vi "PmSetReadoutMode.vi"(8 "error in (no error)":errorcluster, 10 "Readout Mode":T1(ring)=enum."Speed (8-bit)", 11 "Camera in":refnum<class "Camera.lvclass">) -> (0 "error out":errorcluster, 3 "Camera out":refnum<class "Camera.lvclass">)   [LabVIEW 2023, in "Photometrics Camera.lvlib"]
uses:
  Photometrics Camera.lvlib
  Users/Public/Documents/Photometrics/TPM-LabVIEWSamples BETA/TPM LabVIEW adapter/Camera/Camera.lvclass
  Users/Public/Documents/Photometrics/TPM-LabVIEWSamples BETA/TPM LabVIEW adapter/SDK/Controls/Error list.ctl
  C:/Users/Public/Documents/Photometrics/TPM-LabVIEWSamples BETA/TPM LabVIEW adapter/Dependencies/PVCamNET.dll
  Users/Public/Documents/Photometrics/TPM-LabVIEWSamples BETA/TPM LabVIEW adapter/Dependencies/PVCamNET.dll
panel:
  out "index":i32
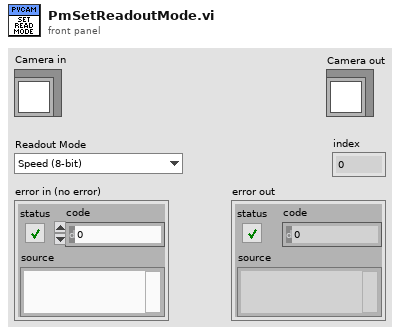
[diagram p1: front panel]
types:
  T1 = enum32{"Sensitivity (12-bit)", "Speed (8-bit)", "Dynamic Range (16-bit)", "Sub-Electron (16-bit)"}
  T2 = typedef "Acquisition Status.ctl" = enum32{"Idle", "Starting", "Acquiring", "Stopping"}
  T3 = typedef "Error list.ctl" = i32
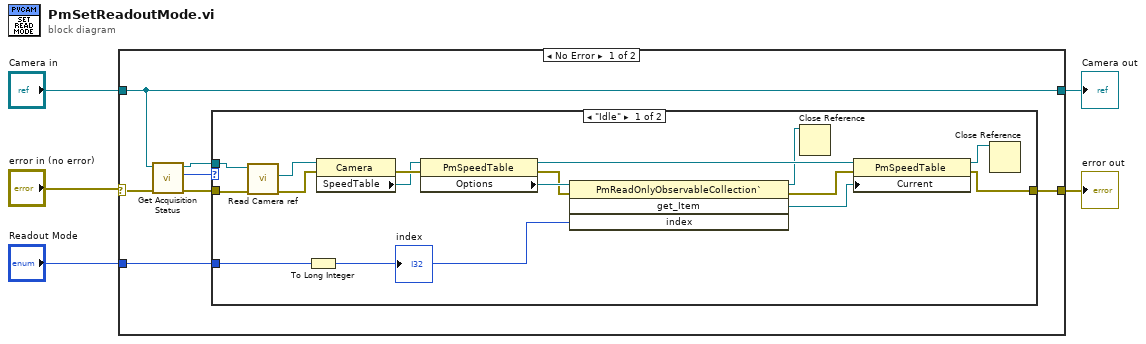
[diagram p0: block diagram]
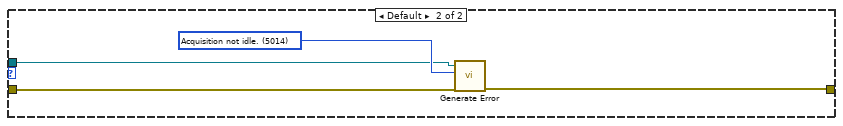
[diagram p2: hidden frame]
diagram:
  n1 = case shown="No Error" "error in (no error)" {
    selector: "error in (no error)" -> [w10 w34]
    tunnel: [w11 w34] -> w5
    tunnel: "Readout Mode" -> [w12 _]
    tunnel: "Camera in" -> [w6 w33]
    tunnel: [w6 w33] -> w1
    frame No Error {
      n2 = call "Get Acquisition Status.vi"("error in (no error)"=w10, "Camera in"=w6) -> ("error out"=w9:errorcluster, "Acquisition Status"=w8:T2, "Camera out"=w7:refnum<class "Camera.lvclass">)  [unwired: 7 in]
      n3 = case shown="\"Idle\"" w8 {
        tunnel: w12 -> [w26 _]
        tunnel: [w24 w29] -> w11
        tunnel: w9 -> [w16 w31]
        tunnel: w7 -> [w15 w30]
        frame "Idle" {
          n4 = call-dynamic "Read Camera ref.vi"("error in (no error)"=w16, "Camera in"=w15) -> ("error out"=w14:errorcluster, "Camera ref"=w13:refnum<k24>)  [unwired: 7 in, 1 out]
          n5 = To Long Integer(number=w26) -> (32bit integer=w25:i32)
          "index" <- w25
          n6 = property class="Camera"(reference=w13, error in=w14) -> (error out=w23:errorcluster, "SpeedTable"=w22:refnum<k24>)  [unwired: 1 out]
          n7 = property class="PmSpeedTable"(reference=w22, error in=w23) -> (reference out=w19:refnum<k24>, error out=w20:errorcluster, "Options"=w21:refnum<k24>)
          n8 = invoke class="PmReadOnlyObservableCollection`" method="get_Item"(reference=w21, error in=w20, "index"=w25) -> (reference out=w18:refnum<k24>, error out=w27:errorcluster, "get_Item"=w28:refnum<k24>)  [unwired: 1 in, 1 out]
          n9 = Close Reference(reference=w18) -> ()  [unwired: 1 in, 1 out]
          n10 = property class="PmSpeedTable"(reference=w19, error in=w27, "Current"=w28) -> (reference out=w17:refnum<k24>, error out=w24:errorcluster)
          n11 = Close Reference(reference=w17) -> ()  [unwired: 1 in, 1 out]
        }
        frame Default {
          w32 = T3 5014 items=["Binning not supported."=5000, "Camera reference is not valid."=5001, "Camera at given index not available."=5002, "Post Processing Index not available."=5003, "Acquisition aborted."=5004, "Acquisition timed out."=5005, "Disk streaming path not valid."=5006, "Enum parameter not available."=5007, "Camera reference not valid."=5008, "Library reference not valid."=5009, "Exceeded the number of supported regions."=5010, "Disk Streaming failed."=5011, "Image saving path not valid."=5012, "Scan Mode parameter not available."=5013, "Acquisition not idle."=5014, "Acquisition idle."=5015] ("PVCAM LabVIEW error")
          n12 = call "Generate Error.vi"("error in (no error)"=w31, "PVCAM LabVIEW error"=w32, "Camera In"=w30) -> ("error out"=w29:errorcluster)  [unwired: 7 in, 1 out]
        }
      }
    }
    frame Error {
    }
  }
  "error out" <- w5
  "Camera out" <- w1
